vi "tonal buttons.vi"(9 "control-level":string, 11 "Material-Scheme in":refnum<class "Material-Scheme.lvclass">) -> (1 "font color":u32(colorbox), 2 "colors array":cluster{"bg":u32, "fg":u32}[](array[cluster]))   [LabVIEW 2021, in "TSC Material Theme.lvlib" / "Material-Scheme.lvclass"]
doc: "application of the TONAL buttons coloring rules\n\nhttps://m3.material.io/components/buttons/specs#31a04913-d070-49c5-9c36-41d551f20096\n\n<b>Code Developed By:</b>\nTechnology Service Corporation\nwww.tsc.com/atcs\n\nDeveloper:\nDaniel Coons"
uses:
  Material-Scheme.lvclass
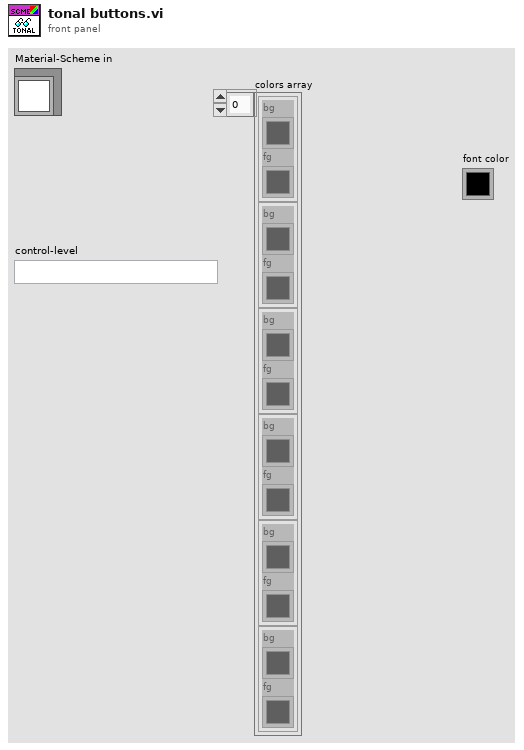
[diagram p1: front panel]
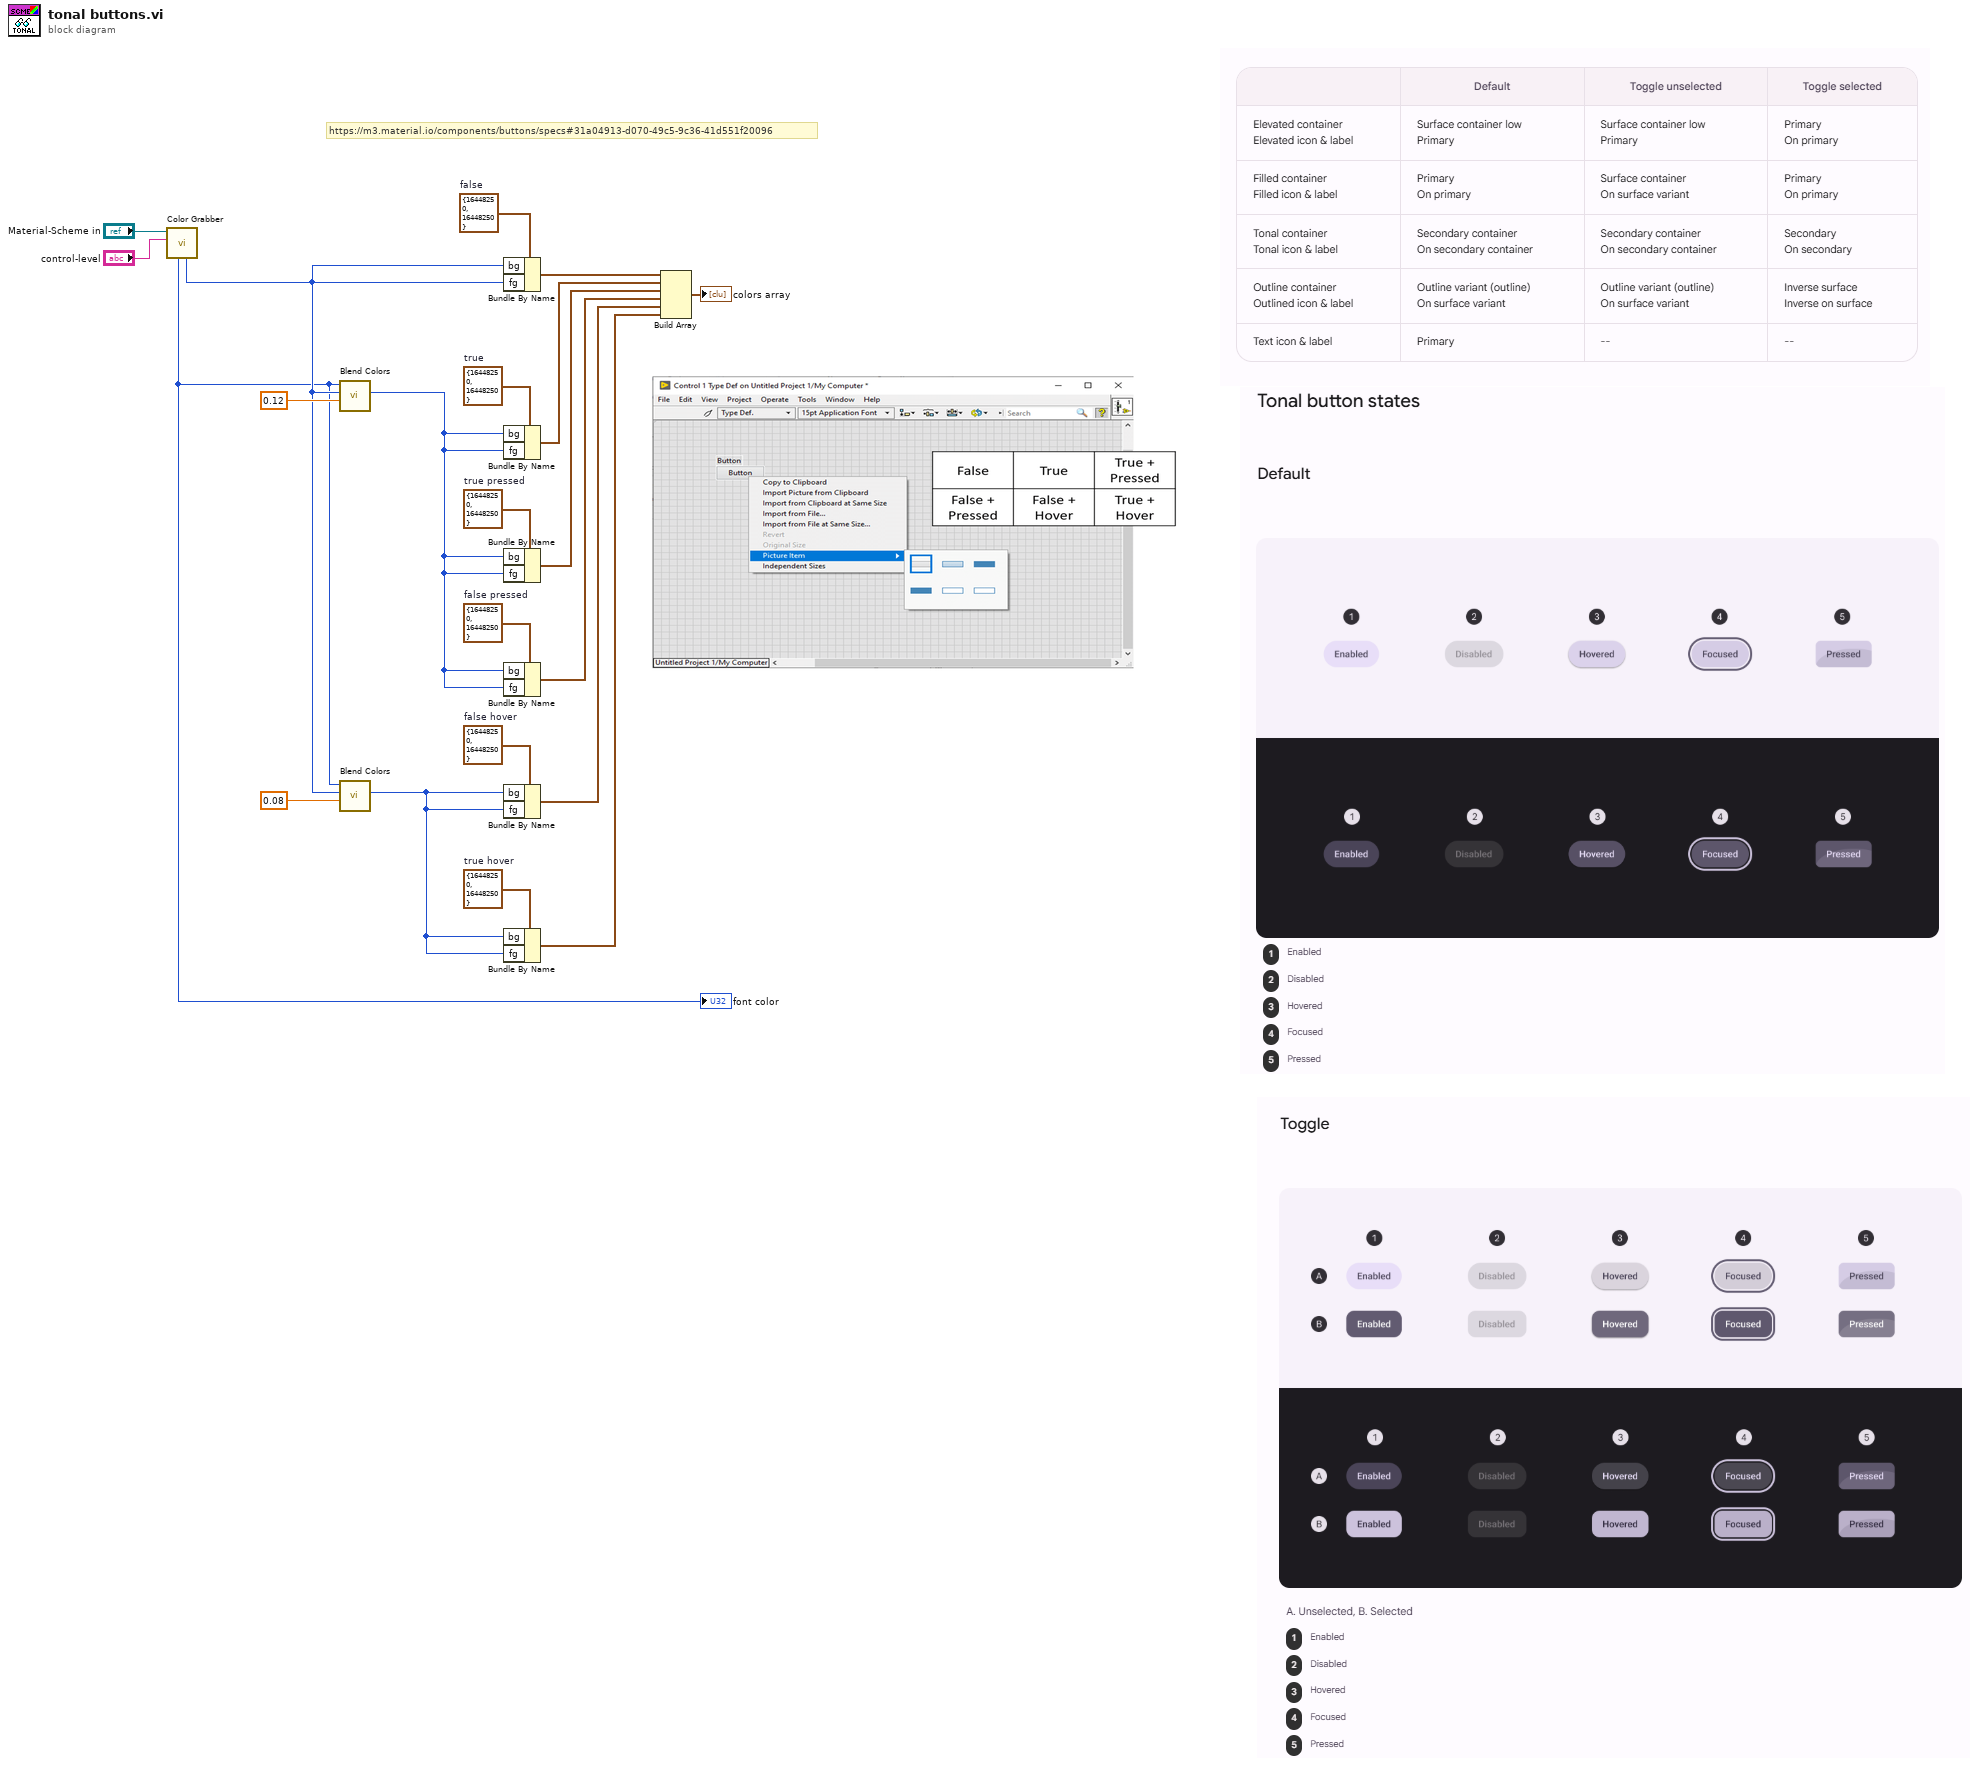
[diagram p0: block diagram]
diagram:
  w16 = cluster{"bg":u32, "fg":u32} {"bg"=16448250, "fg"=16448250}  # true hover
  w17 = cluster{"bg":u32, "fg":u32} {"bg"=16448250, "fg"=16448250}  # false hover
  w18 = cluster{"bg":u32, "fg":u32} {"bg"=16448250, "fg"=16448250}  # false pressed
  w19 = cluster{"bg":u32, "fg":u32} {"bg"=16448250, "fg"=16448250}  # true pressed
  w20 = cluster{"bg":u32, "fg":u32} {"bg"=16448250, "fg"=16448250}  # true
  w21 = cluster{"bg":u32, "fg":u32} {"bg"=16448250, "fg"=16448250}  # false
  # "https://m3.material.io/components/buttons/specs#31a04913-d070-49c5-9c36-41d551f20096"
  n1 = call "Color Grabber.vi"("control-level"="control-level", "Material-Scheme in"="Material-Scheme in") -> ("colorContainer"=w2:u32, "onColorContainer"=w1:u32)  [unwired: 3 in, 5 out]
  "font color" <- w1
  n2 = call "Blend Colors.vi"("blend ratio"=0.12, "onColor"=w2, "Color"=w1) -> ("Modified Color"=w3:u32)  [unwired: 8 in]
  n3 = call "Blend Colors.vi"("blend ratio"=0.08, "onColor"=w2, "Color"=w1) -> ("Modified Color"=w4:u32)  [unwired: 8 in]
  n4 = Bundle By Name(cluster=w21, "bg"=w2, "fg"=w2) -> (w15:cluster{"bg":u32, "fg":u32})
  n5 = Bundle By Name(cluster=w20, "bg"=w3, "fg"=w3) -> (w14:cluster{"bg":u32, "fg":u32})
  n6 = Bundle By Name(cluster=w19, "bg"=w3, "fg"=w3) -> (w13:cluster{"bg":u32, "fg":u32})
  n7 = Bundle By Name(cluster=w18, "bg"=w3, "fg"=w3) -> (w12:cluster{"bg":u32, "fg":u32})
  n8 = Bundle By Name(cluster=w17, "bg"=w4, "fg"=w4) -> (w11:cluster{"bg":u32, "fg":u32})
  n9 = Bundle By Name(cluster=w16, "bg"=w4, "fg"=w4) -> (w10:cluster{"bg":u32, "fg":u32})
  n10 = Build Array(w15, w14, w13, w12, w11, w10) -> (→"colors array":cluster{"bg":u32, "fg":u32}[])
